vi "Set Server Internal UEs.vi"(10 "Server Internal UEs":T1, 11 "OOP Server in":refnum<class "Ex1_server.lvclass">) -> (3 "OOP Server out":refnum<class "Ex1_server.lvclass">)   [LabVIEW 2019, in "Ex1_server.lvlib" / "Ex1_server.lvclass"]
uses:
  Ex1_server.lvclass
  typeDefs/Server Internal UEs.ctl
  typeDefs/Server Internal Message.ctl
  Ex1_server.lvclass/Ex1_server.ctl
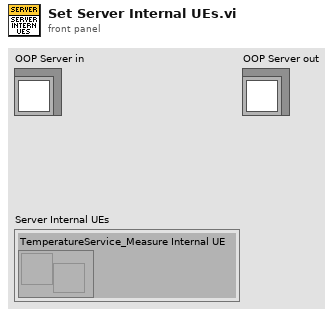
[diagram p1: front panel]
types:
  T1 = typedef "Ex1_server.lvlib/Ex1_server.lvclass/Server Internal UEs.ctl" = cluster{"TemperatureService_Measure Internal UE":refnum<user-event>}
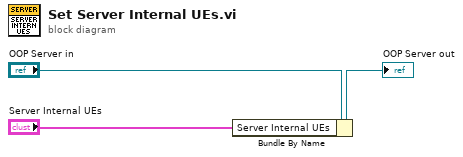
[diagram p0: block diagram]
diagram:
  n1 = Bundle By Name(cluster="OOP Server in", "Server Internal UEs"="Server Internal UEs") -> (→"OOP Server out":refnum<class "Ex1_server.lvclass">)
